vi "Shallow Copy Priv.vi"(0 "Tree Dictionary In":variant, 5 "Unique ID":string, 11 "error in":errorcluster) -> (4 "Tree Dictionary Out":variant, 8 "ID":string, 15 "error out":errorcluster)   [LabVIEW 2017, in "Tree API.lvlib" / "Tree.lvclass"]
uses:
  Tree.lvclass
  Typedefs/Tree Cluster.ctl
  Tree Data/Tree Data.lvclass
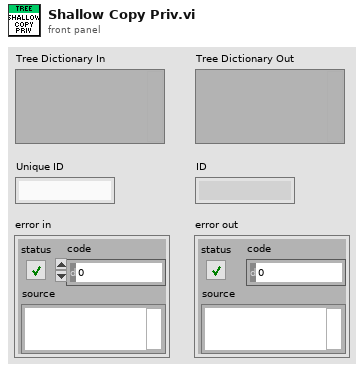
[diagram p1: front panel]
types:
  T1 = typedef "Tree API.lvlib/Tree.lvclass/Tree Cluster.ctl" = cluster{"Unique ID":string, "Parent ID":string, "Child IDs":string[], "Name":string, "MetaData":string, "Data IDs":string[]}
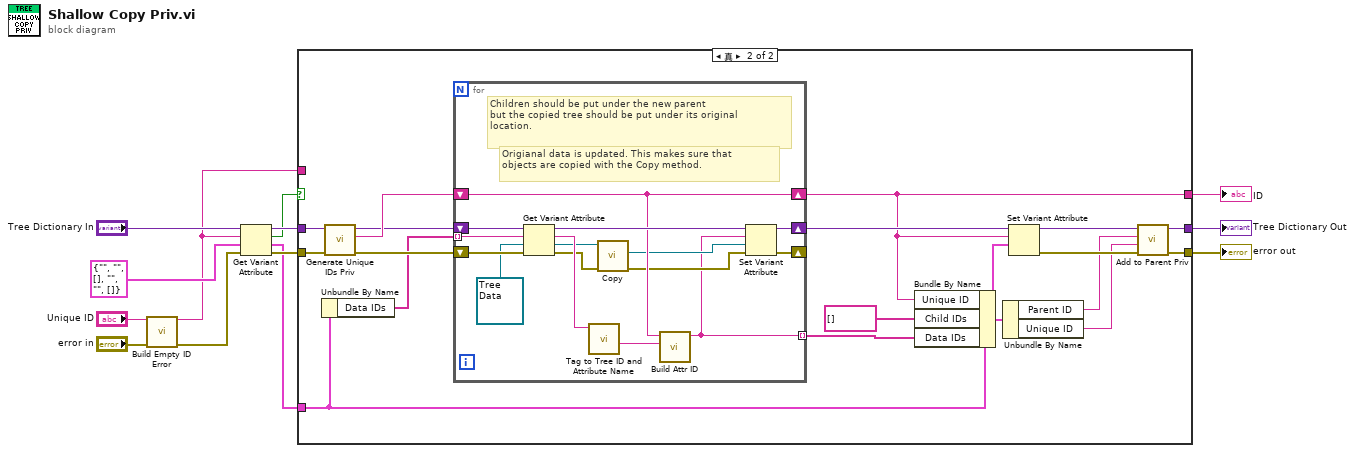
[diagram p0: block diagram]
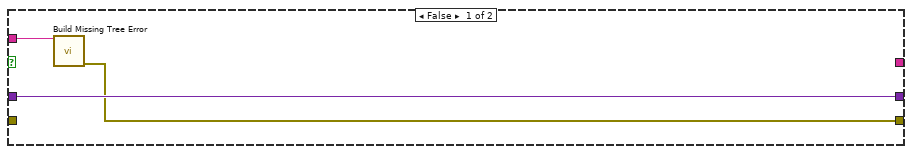
[diagram p2: hidden frame]
diagram:
  n1 = call "Build Empty ID Error.vi"("Unique ID"="Unique ID", "Error In"="error in") -> ("Unique ID Out"=w2:string, "Error Out"=w1:errorcluster)  [unwired: 12 in]
  n2 = Get Variant Attribute(Variant="Tree Dictionary In", name=w2, default value (empty Variant)=T1 {"Unique ID"="", "Parent ID"="", "Child IDs"=[], "Name"="", "MetaData"="", "Data IDs"=[]} ("Cluster of class private data"), error in=w1) -> (duplicate Variant=w9:variant, found=w7:bool, value=w8:T1, error out=w10:errorcluster)
  n3 = case shown="真" w7 {
    tunnel: w8 -> [_ w33]
    tunnel: w9 -> [w16 w24]
    tunnel: w10 -> [_ w23]
    tunnel: [w14 w30] -> w13
    tunnel: [w16 w29] -> w12
    tunnel: w2 -> [w15 _]
    tunnel: [_ w18] -> w6
    frame False {
      n4 = call "Build Missing Tree Error.vi"("Unique ID"=w15) -> ("Error Out"=w14:errorcluster)  [unwired: 14 in]
    }
    frame True {
      n5 = Unbundle By Name(w33) -> ("Data IDs"=w19:string[])
      n6 = call "Generate Unique IDs Priv.vi"("Error In"=w23, "Tree Dictionary"=w24) -> ("Error Out"=w20:errorcluster, "First ID"=w22:string, "Tree Dictionary Out"=w21:variant)  [unwired: 6 in, 1 out]
      n7 = for {
        shift-right: [w41] -> _
        shift-left: w20 -> [w47]
        shift-right: [w42] -> w25
        shift-left: w21 -> [w48]
        tunnel: w19 -> [w45] mode=indexing
        shift-right: [w38] -> w18
        shift-left: w22 -> [w38]
        tunnel: [w35] -> w17 mode=indexing
        # "Children should be put under the new parent\nbut the copied tree should be put under its original\nlocation."
        # "Origianal data is updated. This makes sure that\nobjects are copied with the Copy method."
        n8 = Get Variant Attribute(Variant=w48, name=w45, default value (empty Variant)=refnum<class "Tree Data.lvclass"> refnum ("Tree API.lvlib:Tree Data.lvclass"), error in=w47) -> (duplicate Variant=w43:variant, value=w44:refnum<class "Tree Data.lvclass">, error out=w40:errorcluster)  [unwired: 1 out]
        n9 = call "Tag to Tree ID and Attribute Name.vi"("Tag"=w45) -> ("Attribute Name"=w39:string)  [unwired: 8 in, 2 out]
        n10 = call-dynamic "Copy.vi"("Error In"=w40, "Tree Data"=w44) -> ("Error Out"=w36:errorcluster, "Copy"=w37:refnum<class "Tree Data.lvclass">)  [unwired: 8 in]
        n11 = call "Build Attr ID.vi"("Attr Name"=w39, "Unique ID"=w38) -> ("Attr ID Out"=w35:string)  [unwired: 9 in]
        n12 = Set Variant Attribute(Variant=w43, name=w35, value=w37, error in=w36) -> (Variant out=w42:variant, error out=w41:errorcluster)  [unwired: 1 out]
      }
      n13 = Bundle By Name(cluster=w33, "Unique ID"=w18, "Child IDs"=string[] [], "Data IDs"=w17) -> (w28:T1)
      n14 = Unbundle By Name(w28) -> ("Parent ID"=w27:string, "Unique ID"=w26:string)
      n15 = Set Variant Attribute(Variant=w25, name=w18, value=w28) -> (Variant out=w32:variant, error out=w31:errorcluster)  [unwired: 1 in, 1 out]
      n16 = call "Add to Parent Priv.vi"("Error In"=w31, "Unique ID"=w26, "Parent ID"=w27, "Tree Dictionary"=w32) -> ("Error Out"=w30:errorcluster, "Tree Dictionary Out"=w29:variant)  [unwired: 6 in]
    }
  }
  "error out" <- w13
  "Tree Dictionary Out" <- w12
  "ID" <- w6
